vi "labview调用matlab 1.vi"() -> ()   [LabVIEW 2014]
panel:
  out "?":string
  in  "高速主轴不平衡振动识别":bool
  in  "高速主轴不平衡振动行为分析":bool
  in  "高速主轴系统有限元动力学建模":bool
  in  "角接触球轴承有限元动力学建模":bool
  # "高速主轴不平衡振动行为分析及其抑制方法研究软件系统"
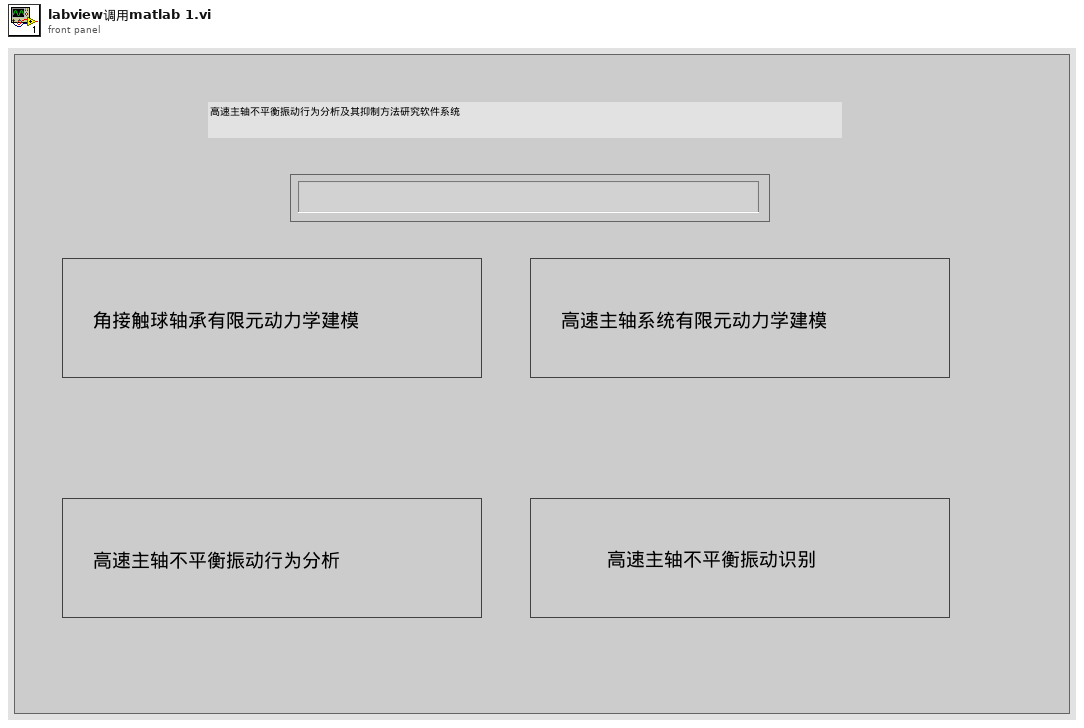
[diagram p1: front panel]
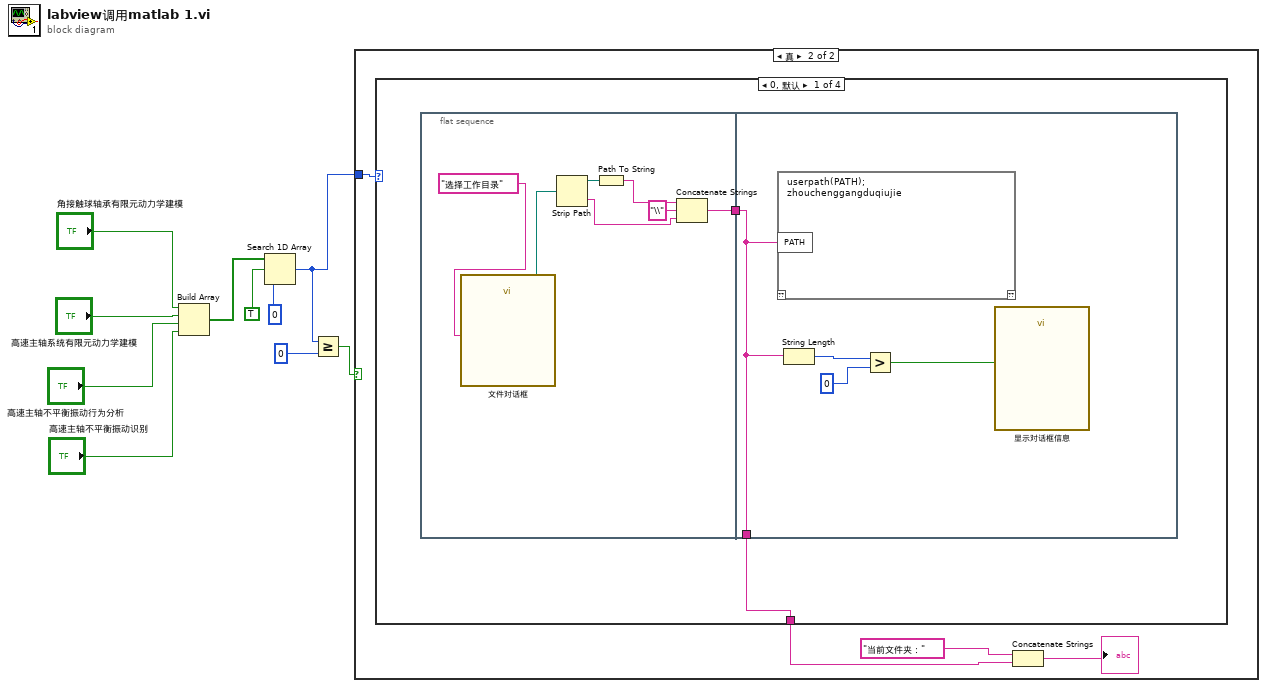
[diagram p0: block diagram]
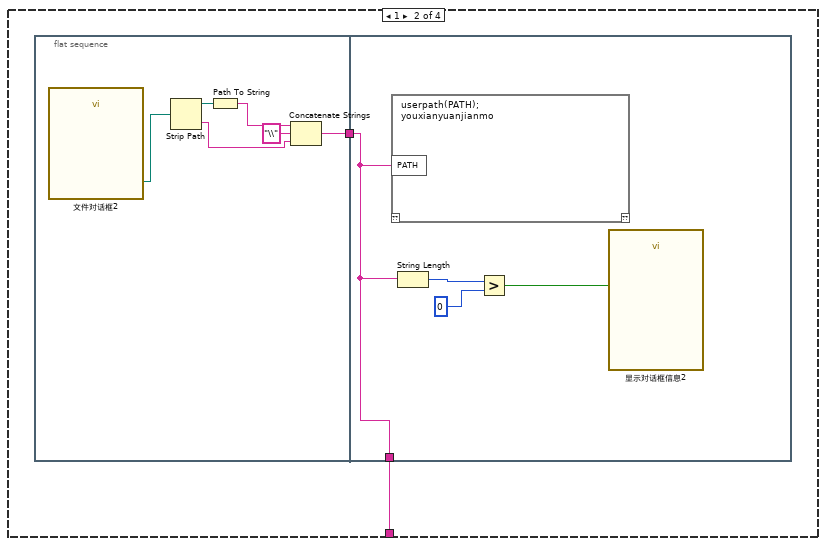
[diagram p3: hidden frame]
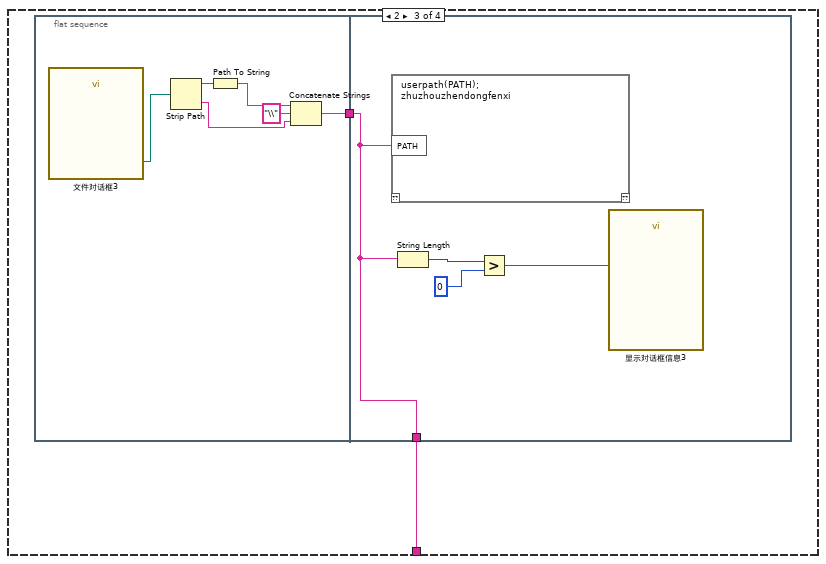
[diagram p4: hidden frame]
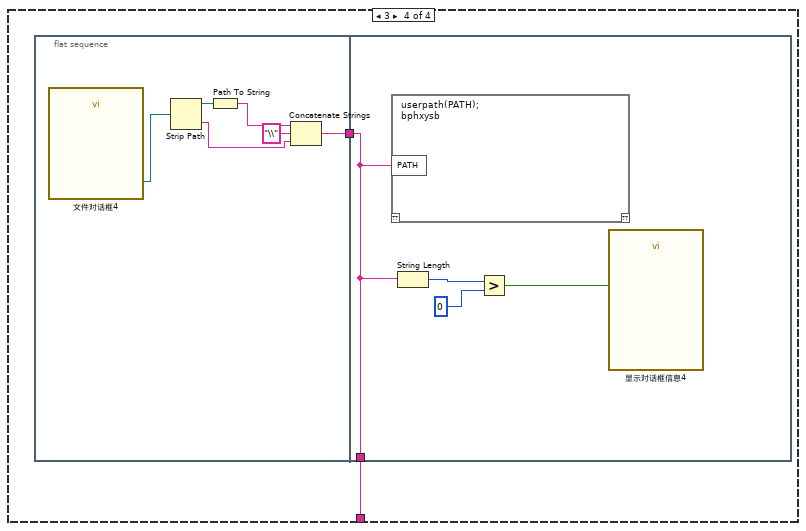
[diagram p5: hidden frame]
diagram:
  n1 = Build Array("角接触球轴承有限元动力学建模", "高速主轴系统有限元动力学建模", "高速主轴不平衡振动行为分析", "高速主轴不平衡振动识别") -> (w6:bool[])
  n2 = Search 1D Array(1D array=w6, element=TRUE, start index (0)=0 ("开始索引(0)")) -> (index of element=w3:i32)
  n3 = Greater Or Equal?(x=w3, y=0 ("开始索引(0)")) -> (x >= y?=w1:bool)
  n4 = case shown="真" w1 {
    tunnel: w3 -> [_ w14]
    frame False {
    }
    frame True {
      n5 = case shown="0, 默认" w14 {
        tunnel: [w15 w28 w40 w52] -> w11
        frame 0, Default {
          n6 = flat-sequence {
            tunnel: [w18] -> w16
            tunnel: w16 -> [w24]
            tunnel: [w24] -> w15
            frame #0 {
              n7 = call "文件对话框"("prompt"="选择工作目录") -> ("selected path"=w23:path)  [unwired: 11 in, 3 out]
              n8 = Strip Path(path=w23) -> (stripped path=w20:path, name=w19:string)
              n9 = Path To String(path=w20) -> (string=w22:string)
              n10 = Concatenate Strings(w22, "\\" ("字符串"), w19) -> (w18:string)
            }
            frame #1 {
              n11 = script code="userpath(PATH);\nzhouchenggangduqiujie"("PATH"=w24) -> ()  [unwired: 1 in, 1 out]
              n12 = String Length(string=w24) -> (length=w27:i32)
              n13 = Greater?(x=w27, y=0) -> (0:w25:bool)
              n14 = call "显示对话框信息"("Enable"=w25) -> ()  [unwired: 9 in, 2 out]
            }
          }
        }
        frame 1 {
          n15 = flat-sequence {
            tunnel: [w30] -> w29
            tunnel: w29 -> [w36]
            tunnel: [w36] -> w28
            frame #0 {
              n16 = call "文件对话框2"() -> ("selected path"=w35:path)  [unwired: 12 in, 3 out]
              n17 = Strip Path(path=w35) -> (stripped path=w32:path, name=w31:string)
              n18 = Path To String(path=w32) -> (string=w34:string)
              n19 = Concatenate Strings(w34, "\\" ("字符串"), w31) -> (w30:string)
            }
            frame #1 {
              n20 = script code="userpath(PATH);\nyouxianyuanjianmo"("PATH"=w36) -> ()  [unwired: 1 in, 1 out]
              n21 = String Length(string=w36) -> (length=w39:i32)
              n22 = Greater?(x=w39, y=0) -> (0:w37:bool)
              n23 = call "显示对话框信息2"("Enable"=w37) -> ()  [unwired: 9 in, 2 out]
            }
          }
        }
        frame 2 {
          n24 = flat-sequence {
            tunnel: [w42] -> w41
            tunnel: w41 -> [w48]
            tunnel: [w48] -> w40
            frame #0 {
              n25 = call "文件对话框3"() -> ("selected path"=w47:path)  [unwired: 12 in, 3 out]
              n26 = Strip Path(path=w47) -> (stripped path=w44:path, name=w43:string)
              n27 = Path To String(path=w44) -> (string=w46:string)
              n28 = Concatenate Strings(w46, "\\" ("字符串"), w43) -> (w42:string)
            }
            frame #1 {
              n29 = script code="userpath(PATH);\nzhuzhouzhendongfenxi"("PATH"=w48) -> ()  [unwired: 1 in, 1 out]
              n30 = String Length(string=w48) -> (length=w51:i32)
              n31 = Greater?(x=w51, y=0) -> (0:w49:bool)
              n32 = call "显示对话框信息3"("Enable"=w49) -> ()  [unwired: 9 in, 2 out]
            }
          }
        }
        frame 3 {
          n33 = flat-sequence {
            tunnel: [w54] -> w53
            tunnel: w53 -> [w60]
            tunnel: [w60] -> w52
            frame #0 {
              n34 = call "文件对话框4"() -> ("selected path"=w59:path)  [unwired: 12 in, 3 out]
              n35 = Strip Path(path=w59) -> (stripped path=w56:path, name=w55:string)
              n36 = Path To String(path=w56) -> (string=w58:string)
              n37 = Concatenate Strings(w58, "\\" ("字符串"), w55) -> (w54:string)
            }
            frame #1 {
              n38 = script code="userpath(PATH);\nbphxysb"("PATH"=w60) -> ()  [unwired: 1 in, 1 out]
              n39 = String Length(string=w60) -> (length=w63:i32)
              n40 = Greater?(x=w63, y=0) -> (0:w61:bool)
              n41 = call "显示对话框信息4"("Enable"=w61) -> ()  [unwired: 9 in, 2 out]
            }
          }
        }
      }
      n42 = Concatenate Strings("当前文件夹：" ("字符串"), w11) -> (→"?":string)
    }
  }
